vi "UI - Read Stream from RT.vi"(11 "Message Queue":refnum<queue>) -> (0 "error out":errorcluster, 2 "Message Received?":bool, 3 "dup Message Queue":refnum<queue>)   [LabVIEW 2018]
uses:
  Message Queue/Message Cluster.ctl
  Globals/Global - UI Stream and Variable Connections.vi
  Message Queue/Message Queue.lvlib
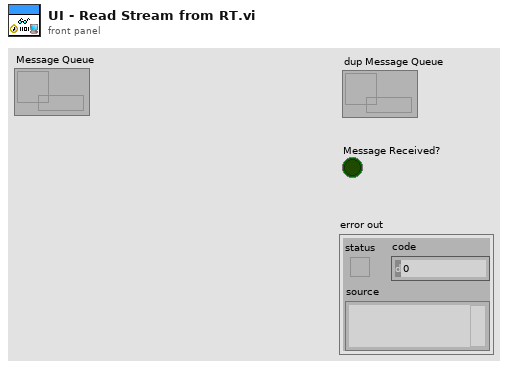
[diagram p1: front panel]
types:
  T1 = typedef "Message Queue.lvlib/Message Cluster.ctl" = cluster{"Message":string, "Message Data":variant}
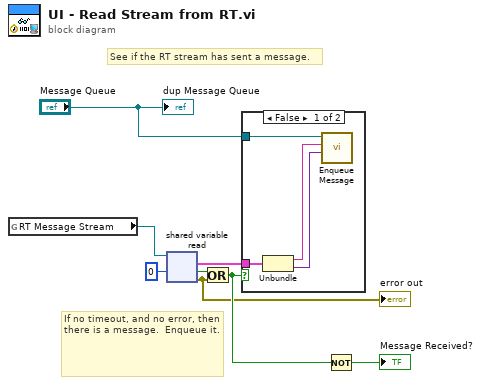
[diagram p0: block diagram]
diagram:
  # "If no timeout, and no error, then there is a message.  Enqueue it."
  # "See if the RT stream has sent a message."
  n1 = global read "Global - UI Stream and Variable Connections.vi" "RT Message Stream"() -> (w3:refnum<k21>)
  n2 = shared-variable-read(w3, 0 ("timeout ms (-1)")) -> (w5:errorcluster, w8:bool, w6:T1)  [unwired: 1 in, 1 out]
  "error out" <- w5
  n3 = Or(x=w8, y=w5) -> (x .or. y?=w7:bool)
  n4 = case shown="False" w7 {
    tunnel: w6 -> [w11 _]
    tunnel: "Message Queue" -> [w12 _]
    frame False {
      n5 = Unbundle(w11) -> ("Message"=w10:string, "Message Data"=w9:variant)
      n6 = call "Enqueue Message.vi"("Message Data"=w9, "Message"=w10, "Message Queue"=w12) -> ()  [unwired: 7 in, 2 out]
    }
    frame True {
    }
  }
  n7 = Not(x=w7) -> (.not. x?=→"Message Received?":bool)
  "dup Message Queue" <- "Message Queue"
